vi "autoCoag.vi"(6 "state":T2, 7 "current time":timestamp, 8 "error in (no error)":errorcluster, 10 "data input":T1) -> (0 "error out":errorcluster, 2 "total HRT":dbl, 4 "HRT (s)":dbl)   [LabVIEW 2019]
uses:
  state.ctl
  coag model data.ctl
  ini.ctl
  Sensor buffer command.ctl
  file paths.ctl
  data cluster.ctl
  <vilib>/Utility/config.llb/Read Key (String).vi
  <vilib>/Utility/config.llb/Write Key (String).vi
  <vilib>/Utility/config.llb/NI_LVConfig.lvlib
panel:
  out "length":i32
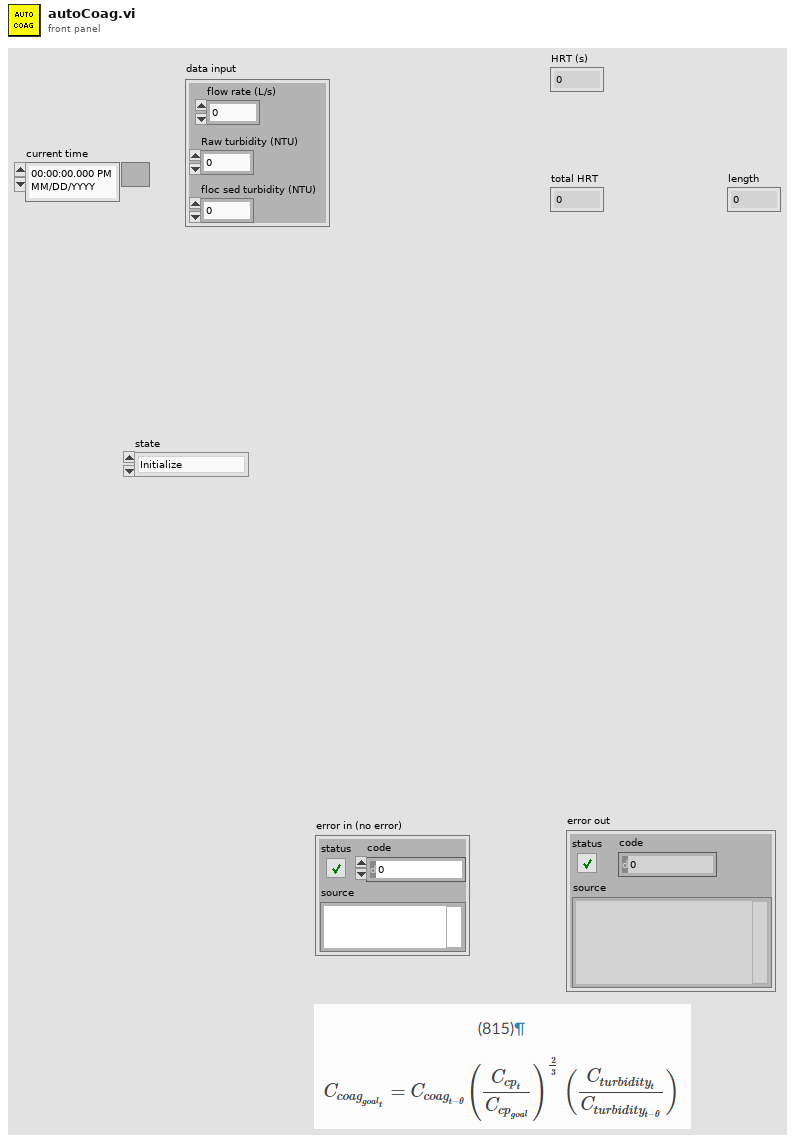
[diagram p1: front panel]
types:
  T1 = typedef "coag model data.ctl" = cluster{"flow rate (L/s)":dbl, "Raw turbidity (NTU)":dbl, "floc sed turbidity (NTU)":dbl}
  T2 = typedef "state.ctl" = enum16{"Initialize", "Process data", "Close"}
  T3 = typedef "ini.ctl" = enum16{"write", "read"}
  T4 = typedef "file paths.ctl" = enum16{"read paths", "close"}
  T5 = typedef "Sensor buffer command.ctl" = enum16{"set buffer size", "write", "refill buffer", "read recent", "read all", "read at delta HRT", "clear"}
  T6 = typedef "data cluster.ctl" = cluster{"floc sed turbidity (NTU)":dbl, "Raw turbidity (NTU)":dbl, "flow rate (L/s)":dbl, "time":timestamp, "Cumulative HRT":dbl, "Coag dose (mg/L)":dbl, "DOM coag demand (mg/L)":dbl, "DOM in range":bool}
  T7 = typedef "setpoints.ctl" = cluster{"graph data interval (s)":sgl, "sludge flow [L/s]":dbl, "plant flow [L/s]":dbl, "Plant Flow PID ":cluster{"proportional gain (Kc)":dbl, "integral time (Ti, min)":dbl, "derivative time (Td, min)":dbl}, "Sludge PID ":cluster{"proportional gain (Kc)":dbl, "integral time (Ti, min)":dbl, "derivative time (Td, min)":dbl}, "backwash":T8, "Coagulant":T9}
  T8 = typedef "backwash.ctl" = cluster{"Filtered quality target [NTU]":dbl, "min filtration time [s]":dbl, "Ripen time [s]":dbl}
  T9 = typedef "coag.ctl" = cluster{"flocculator volume (L)":dbl, "clarifier volume (L)":dbl, "dose updates per response delay":u16, "target clarified turbidity (NTU)":dbl, "Coagulant mode":T10, "Coag dose [mg/L]":dbl, "pump mL/rev":dbl, "clarifier flow [L/s]":dbl, "min Coag dose [mg/L]":dbl, "max Coag dose [mg/L]":dbl, "Steps":u16, "HRT response delay":u32, "kpf":dbl, "DOM coag demand [mg/L]":dbl, "min DOM coag demand [mg/L]":dbl, "max DOM coag demand [mg/L]":dbl}
  T10 = typedef "model type.ctl" = enum16{"manual", "ramp", "simple corrector"}
  T11 = typedef "NI_LVConfig.lvlib/Config Data RefNum.ctl" = refnum<k1>
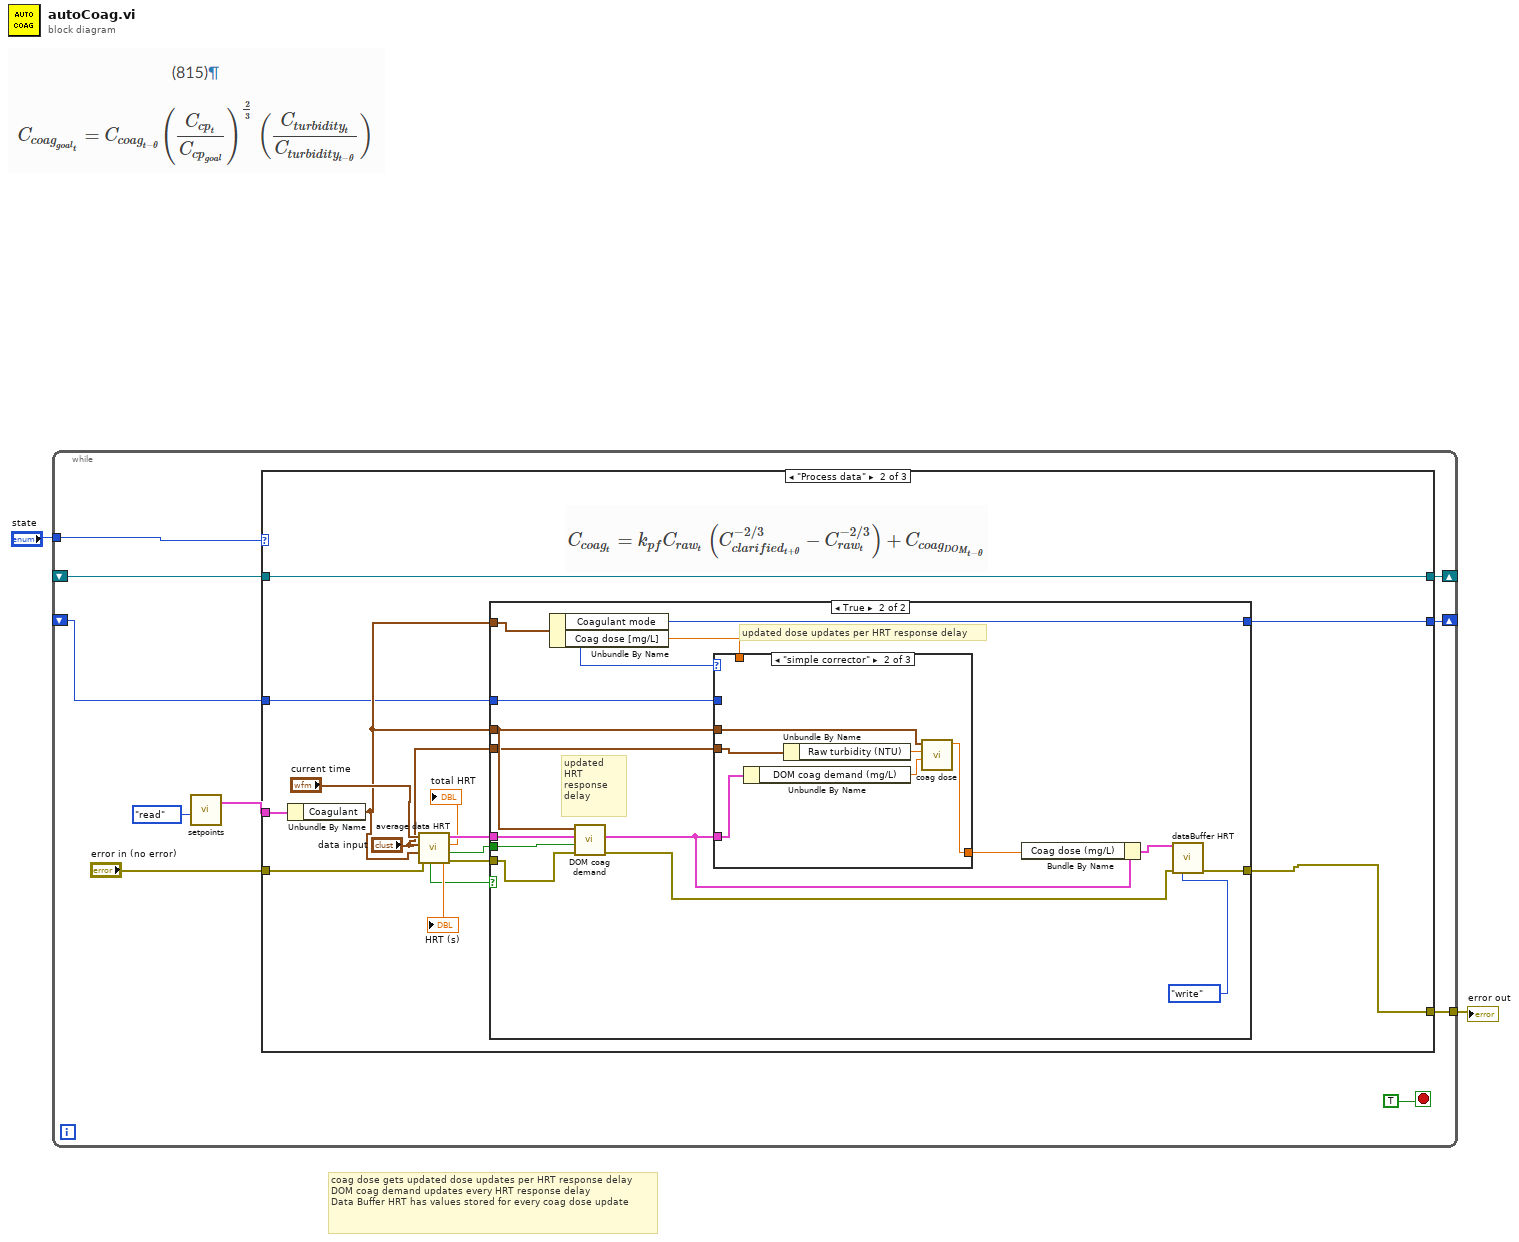
[diagram p0: block diagram]
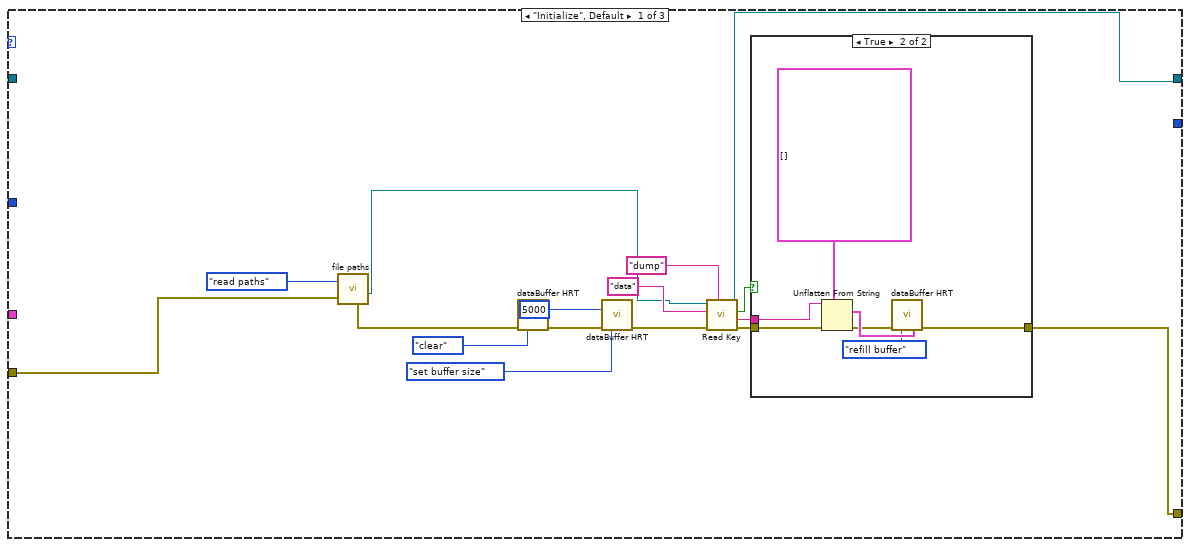
[diagram p2: hidden frame]
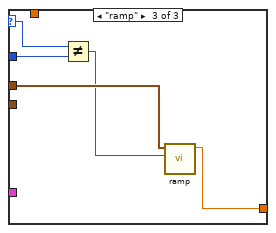
[diagram p6: hidden frame]
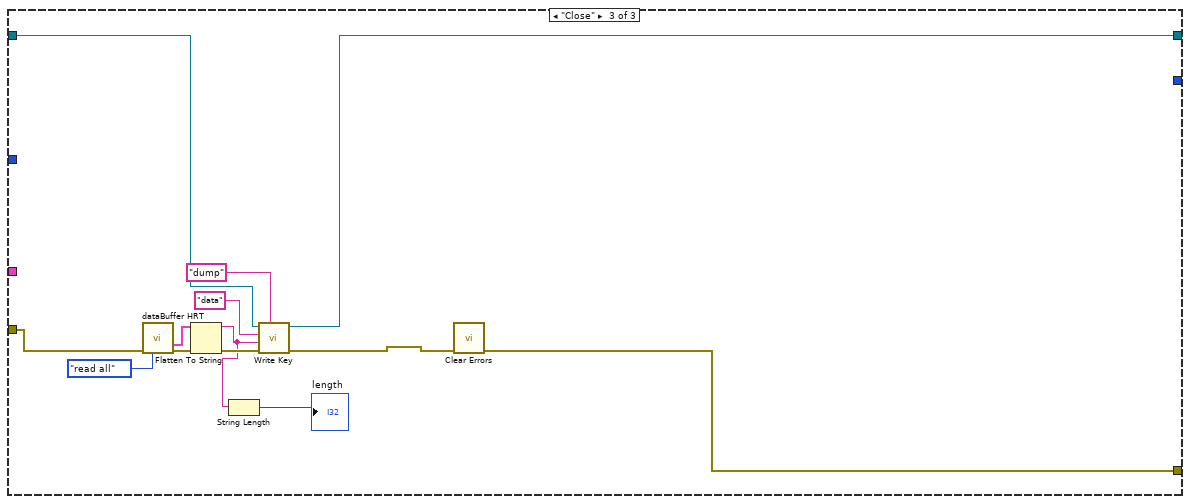
[diagram p7: hidden frame]
diagram:
  # "coag dose gets updated dose updates per HRT response delay\nDOM coag demand updates every HRT response delay\nData Buffer HRT has values stored for every coag dose update"
  n1 = while {
    tunnel: "state" -> [w11]
    shift-right: [w10] -> _
    shift-left: _ -> [w9]
    tunnel: [w8] -> w1
    shift-right: [w4] -> _
    shift-left: _ -> [w3]
    stop <- TRUE stop-if-true
    n2 = call "setpoints.vi"("ini"=ini."read") -> ("Setpoints out"=w6:T7)  [unwired: 9 in, 1 out]
    n3 = case shown="\"Process data\"" w11 {
      tunnel: [w15 w51 w80] -> w10
      tunnel: w9 -> [_ w51 w91]
      tunnel: w6 -> [_ w45 _]
      tunnel: [w16 w39 w82] -> w8
      tunnel: "error in (no error)" -> [w18 w49 w89]
      tunnel: [_ w42 _] -> w4
      tunnel: w3 -> [_ w41 _]
      frame "Initialize", Default {
        n4 = call "file paths.vi"("error in (no error)"=w18, "file path control"=file_paths."read paths") -> ("ini"=w19:T11, "error out"=w17:errorcluster)  [unwired: 6 in, 2 out]
        n5 = call "dataBuffer HRT.vi"("error in (no error)"=w17, "command"=Sensor_buffer_command."clear") -> ("error out"=w26:errorcluster)  [unwired: 8 in, 5 out]
        n6 = call "dataBuffer HRT.vi"("max array size"=u16 5000, "error in (no error)"=w26, "command"=Sensor_buffer_command."set buffer size") -> ("error out"=w23:errorcluster)  [unwired: 7 in, 5 out]
        n7 = call-poly <vilib>:"Read Key.vi"("section"="dump", "error in (no error)"=w23, "key"="data", "refnum"=w19) -> ("error out"=w22:errorcluster, "value"=w21:string, "found?"=w20:bool, "refnum out"=w15:T11)  [unwired: 4 in]
        n8 = case shown="True" w20 {
          tunnel: w22 -> [w29 w36]
          tunnel: w21 -> [_ w35]
          tunnel: [w29 w30] -> w16
          frame False {
          }
          frame True {
            n9 = Unflatten From String(type=T6[] [] ("all data out"), binary string=w35, error in (no error)=w36) -> (value=w33:T6[], error out=w31:errorcluster)  [unwired: 2 in, 1 out]
            n10 = call "dataBuffer HRT.vi"("error in (no error)"=w31, "command"=Sensor_buffer_command."refill buffer", "all data in"=w33) -> ("error out"=w30:errorcluster)  [unwired: 7 in, 5 out]
          }
        }
      }
      frame "Process data" {
        n11 = Unbundle By Name(w45) -> ("Coagulant"=w43:T9)
        n12 = call "average data HRT.vi"("error in (no error)"=w49, "Coagulant"=w43, "data input"="data input", "seconds since 1Jan1904"="current time") -> ("error out"=w48:errorcluster, "update DOM demand"=w37:bool, "total HRT"=→"total HRT":dbl, "averaged data"=w50:T6, "HRT (s)"=→"HRT (s)":dbl, "update coag dose"=w38:bool)  [unwired: 2 in]
        n13 = case shown="True" w38 {
          tunnel: w50 -> [_ w65]
          tunnel: w48 -> [w52 w54]
          tunnel: [w52 w58] -> w39
          tunnel: w43 -> [_ w67]
          tunnel: w43 -> [_ w64]
          tunnel: [_ w61] -> w42
          tunnel: w41 -> [_ w60]
          tunnel: "data input" -> [_ w59]
          tunnel: w37 -> [_ w53]
          frame False {
          }
          frame True {
            # "updated HRT response delay"
            # "updated dose updates per HRT response delay"
            n14 = Unbundle By Name(w67) -> ("Coagulant mode"=w61:T10, "Coag dose [mg/L]"=w66:dbl)
            n15 = call "DOM coag demand.vi"("error in (no error)"=w54, "update DOM coag demand"=w53, "averaged data"=w65, "Coagulant"=w64) -> ("error out"=w57:errorcluster, "averaged data with coag demand"=w63:T6)  [unwired: 4 in, 2 out]
            n16 = case shown="\"simple corrector\"" w61 {
              selector: w61 -> [_ _ w76]
              tunnel: [w68 w69 w79] -> w62
              tunnel: w66 -> [w68 _ _]
              tunnel: w64 -> [_ w70 w78]
              tunnel: w63 -> [_ w74 _]
              tunnel: w60 -> [_ _ w77]
              tunnel: w59 -> [_ w73 _]
              frame "manual", Default {
              }
              frame "simple corrector" {
                n17 = Unbundle By Name(w74) -> ("DOM coag demand (mg/L)"=w72:dbl)
                n18 = Unbundle By Name(w73) -> ("Raw turbidity (NTU)"=w71:dbl)
                n19 = call "coag dose.vi"("DOM coag demand (mg/L)"=w72, "raw water turbidity (NTU)"=w71, "Coagulant"=w70) -> ("coag dose (mg/L)"=w69:dbl)  [unwired: 8 in]
              }
              frame "ramp" {
                n20 = Not Equal?(x=w76, y=w77) -> (x != y?=w75:bool)
                n21 = call "ramp.vi"("reset"=w75, "Coagulant"=w78) -> ("Coag dose"=w79:dbl)  [unwired: 9 in]
              }
            }
            n22 = Bundle By Name(cluster=w63, "Coag dose (mg/L)"=w62) -> (w55:T6)
            n23 = call "dataBuffer HRT.vi"("averaged data"=w55, "error in (no error)"=w57, "command"=Sensor_buffer_command."write") -> ("error out"=w58:errorcluster)  [unwired: 7 in, 5 out]
          }
        }
      }
      frame "Close" {
        n24 = call "dataBuffer HRT.vi"("error in (no error)"=w89, "command"=Sensor_buffer_command."read all") -> ("all data out"=w90:T6[], "error out"=w88:errorcluster)  [unwired: 8 in, 4 out]
        n25 = Flatten To String(anything=w90, error in (no error)=w88) -> (data string=w84:string, error out=w87:errorcluster)  [unwired: 2 in, 1 out]
        n26 = String Length(string=w84) -> (length=→"length":i32)
        n27 = call-poly <vilib>:"Write Key.vi"("section"="dump", "error in (no error)"=w87, "value"=w84, "key"="data", "refnum"=w91) -> ("error out"=w81:errorcluster, "refnum out"=w80:T11)  [unwired: 4 in, 1 out]
        n28 = call <vilib>:"Clear Errors.vi"("error in (no error)"=w81) -> ("error out"=w82:errorcluster)  [unwired: 5 in, 1 out]
      }
    }
  }
  "error out" <- w1
